vi "check config on connection.vi"() -> (3 "config data out":T18={"Message"={"Parameters"={"FPGA Ref"=refnum, "configID"=0, "activeChannels"=[]}, "Variables"={"RT Status"={"Comms loop"=FALSE, "scheduler loop"=FALSE, "data process loop"=FALSE, "FIFO loop"=FALSE, "Command Stream"=FALSE, "Error Stream"=FALSE, "FPGA FIFO"=FALSE, "Data Stream"=FALSE}, "watchdog"=timestamp(0 s since 1904-01-01), "limitsEnabled"=FALSE, "Interlocks"={"gearboxOil"=FALSE, "bearingOil"=FALSE, "gearboxAir"=FALSE}}}, "FIFO"={"Params"={"FPGA ref"=refnum, "Total Channels"=0}, "Variables"={"FIFO wait counter"=0, "FIFO read trigger"=0}}, "Comms data"={"Parameters"={"error writer name"="", "command reader name"="", "error buffer size"=0, "command buffer size"=0, "scanivalveIP"="", "scanivalvePeriod"=0}, "Variables"={"listen schedule"=0, "incident buffer"=[], "command stream"="", "error stream"="", "waiting for command stream connect"=FALSE, "waiting for error stream connect"=FALSE, "scanivalve connection"=refnum, "scanivalveScheduleID"=0, "activeScanivalvePorts"=[], "channelCount"=0}, "scanivalveConfig"={"listS"={"period"=0, "ADtrig"=FALSE, "ScanTrig"=FALSE, "page"=0, "qpkts"=0}, "listC"={"ZC"=FALSE, "unitScan"="", "CvtUnit"=0.0, "bin"=FALSE, "EU"=FALSE}, "listSG"={"Avg1"=0, "FPS1"=0, "SGEnable1"=FALSE}, "activeChannels"={"Chan1"={"101"=FALSE, "102"=FALSE, "103"=FALSE, "104"=FALSE, "109"=FALSE, "110"=FALSE, "111"=FALSE, "112"=FALSE, "201"=FALSE, "202"=FALSE, "203"=FALSE, "204"=FALSE, "209"=FALSE, "210"=FALSE, "211"=FALSE, "212"=FALSE, "301"=FALSE, "302"=FALSE, "303"=FALSE, "304"=FALSE, "309"=FALSE, "310"=FALSE, "311"=FALSE, "312"=FALSE, "401"=FALSE, "402"=FALSE, "403"=FALSE, "404"=FALSE, "409"=FALSE, "410"=FALSE, "411"=FALSE, "412"=FALSE}}}}, "Data processor"={"Parameters"={"FPGA Ref"=refnum, "data stream"={"data writer name"="error writer", "NS write buffer size"=16, "NS Buffer length"=0}, "FIFO Depth"=0, "Channel controls"={"FIFO channel count"=0, "active indices"=[], "active channels"=0, "channelScaling"=[], "scanivalveCount"=0, "channels"=[]}, "safetyChannels"={"oilP"=0, "airP"=0, "water"=0, "channelLimits"=[]}, "speedChannel"=0, "maxSpeedLimit"=0.0, "Torque"={"fixedOffset"=0.0, "filter"=FALSE, "fallingEdge"=FALSE, "swapEncoders"=FALSE}}, "Variables"={"Intermediary buffer"=[], "buffer position"=0, "write loop counter"=0, "NS write trigger"=0, "NS Connection status"=FALSE, "waiting for NS"=FALSE, "labAmbient"={"pressure"=0.0, "temperature"=0.0}, "scanivalvePorts"=[], "scanivalvePressures"=[], "data stream"="", "activeChannelLimitIndex"=[], "runningSpeedLimit"=0.0, "speedChannelIndex"=0, "Interlocks"={"gearboxOil"=FALSE, "bearingOil"=FALSE, "gearboxAir"=FALSE}, "interlockChannels"={"gearboxOil"=0, "bearingOil"=0, "air"=0}, "limitStates"=[]}}})   [LabVIEW 2018]
uses:
  Type Defs/Message loop data.ctl
  Type Defs/FPGA reference.ctl
  Type Defs/RT Status.ctl
  Type Defs/Analogue loop data.ctl
  Communications loop/comms data.ctl
  Type Defs/generic incident.ctl
  ICL-LabVIEW_General/Scanivalve API project/full interface/polymorphic/scanivalveConfig.ctl
  ICL-LabVIEW_General/Scanivalve API project/full interface/listS.ctl
  ICL-LabVIEW_General/Scanivalve API project/full interface/listC.ctl
  ICL-LabVIEW_General/Scanivalve API project/full interface/listSG.ctl
  ICL-LabVIEW_General/Scanivalve API project/full interface/chan1.ctl
  Type Defs/Data processing loop data.ctl
  PC/type defs/channelControl.ctl
  Type Defs/channelScalingTypes.ctl
  Type Defs/scalingMethods.ctl
  ICL-LabVIEW_General/data channels/parent class/Data Channel.lvclass
  PC/type defs/channelLimitControl.ctl
  PC/type defs/limitActions.ctl
  Type Defs/channelConfigFilePath.ctl
  Type Defs/configFilePath.ctl
  <resource>/objmgr/ni.dex.rc
  ICL-LabVIEW_General/Scanivalve API project/Scanivalve API.lvlib
types:
  T1 = typedef "Message loop data.ctl" = cluster{"Parameters":cluster{"FPGA Ref":T2, "configID":u32, "activeChannels":cluster{"index":u16, "name":string}[]}, "Variables":cluster{"RT Status":T3, "watchdog":timestamp, "limitsEnabled":bool, "Interlocks":cluster{"gearboxOil":bool, "bearingOil":bool, "gearboxAir":bool}}}
  T2 = typedef "FPGA reference.ctl" = refnum<k20>
  T3 = typedef "RT Status.ctl" = cluster{"Comms loop":bool, "scheduler loop":bool, "data process loop":bool, "FIFO loop":bool, "Command Stream":bool, "Error Stream":bool, "FPGA FIFO":bool, "Data Stream":bool}
  T4 = typedef "Analogue loop data.ctl" = cluster{"Params":cluster{"FPGA ref":T2, "Total Channels":u32}, "Variables":cluster{"FIFO wait counter":u16, "FIFO read trigger":u32}}
  T5 = typedef "comms data.ctl" = cluster{"Parameters":cluster{"error writer name":string, "command reader name":string, "error buffer size":i32, "command buffer size":i32, "scanivalveIP":string, "scanivalvePeriod":u16}, "Variables":cluster{"listen schedule":u32, "incident buffer":T6[], "command stream":refnum<k21>, "error stream":refnum<k21>, "waiting for command stream connect":bool, "waiting for error stream connect":bool, "scanivalve connection":refnum<k5>, "scanivalveScheduleID":u32, "activeScanivalvePorts":i32[], "channelCount":i16}, "scanivalveConfig":T7}
  T6 = typedef "generic incident.ctl" = cluster{"timestamp":timestamp, "type":string, "Variant":variant}
  T7 = typedef "Scanivalve API.lvlib/scanivalveConfig.ctl" = cluster{"listS":T8, "listC":T9, "listSG":T10, "activeChannels":T11}
  T8 = typedef "Scanivalve API.lvlib/listS.ctl" = cluster{"period":u16, "ADtrig":bool, "ScanTrig":bool, "page":u16, "qpkts":u16}
  T9 = typedef "Scanivalve API.lvlib/listC.ctl" = cluster{"ZC":bool, "unitScan":string, "CvtUnit":dbl, "bin":bool, "EU":bool}
  T10 = typedef "Scanivalve API.lvlib/listSG.ctl" = cluster{"Avg1":u16, "FPS1":u16, "SGEnable1":bool}
  T11 = typedef "Scanivalve API.lvlib/chan1.ctl" = cluster{"Chan1":cluster{"101":bool, "102":bool, "103":bool, "104":bool, "109":bool, "110":bool, "111":bool, "112":bool, "201":bool, "202":bool, "203":bool, "204":bool, "209":bool, "210":bool, "211":bool, "212":bool, "301":bool, "302":bool, "303":bool, "304":bool, "309":bool, "310":bool, "311":bool, "312":bool, "401":bool, "402":bool, "403":bool, "404":bool, "409":bool, "410":bool, "411":bool, "412":bool}}
  T12 = typedef "Data processing loop data.ctl" = cluster{"Parameters":cluster{"FPGA Ref":T2, "data stream":cluster{"data writer name":string, "NS write buffer size":i32, "NS Buffer length":u32}, "FIFO Depth":u32, "Channel controls":cluster{"FIFO channel count":i32, "active indices":i16[], "active channels":i32, "channelScaling":T13[], "scanivalveCount":i32, "channels":refnum<class "Data Channel.lvclass">[]}, "safetyChannels":cluster{"oilP":u16, "airP":u16, "water":u16, "channelLimits":T16[]}, "speedChannel":i32, "maxSpeedLimit":dbl, "Torque":cluster{"fixedOffset":dbl, "filter":bool, "fallingEdge":bool, "swapEncoders":bool}}, "Variables":cluster{"Intermediary buffer":dbl[][], "buffer position":u32, "write loop counter":u16, "NS write trigger":u32, "NS Connection status":bool, "waiting for NS":bool, "labAmbient":cluster{"pressure":dbl, "temperature":dbl}, "scanivalvePorts":u16[], "scanivalvePressures":dbl[], "data stream":refnum<k21>, "activeChannelLimitIndex":u16[], "runningSpeedLimit":dbl, "speedChannelIndex":i32, "Interlocks":cluster{"gearboxOil":bool, "bearingOil":bool, "gearboxAir":bool}, "interlockChannels":cluster{"gearboxOil":i32, "bearingOil":i32, "air":i32}, "limitStates":cluster{"warn":bool, "alarm":bool}[]}}
  T13 = typedef "channelControl.ctl" = cluster{"index":u16, "active":bool, "channelType":T14, "module":u16, "terminal":u16, "channelName":string, "scalingMethod":T15, "scalingParameters":dbl[], "scaledUnits":string, "tempOffset":dbl}
  T14 = typedef "channelScalingTypes.ctl" = enum16{"calculation", "measurement", "scanivalve", "output", "digital"}
  T15 = typedef "scalingMethods.ctl" = enum16{"none", "linear", "thermocouple", "polynomial", "encoder", "RTD"}
  T16 = typedef "channelLimitControl.ctl" = cluster{"channelID":u16, "Enabled":bool, "warnValue":dbl, "limitValue":dbl, "Invert":bool, "limitAction":T17}
  T17 = typedef "limitActions.ctl" = enum16{"stop", "shutdown", "ignore"}
  T18 = cluster{"Message":T1, "FIFO":T4, "Comms data":T5, "Data processor":T12}
  T19 = typedef "configFilePath.ctl" = path
  T20 = typedef "channelConfigFilePath.ctl" = path
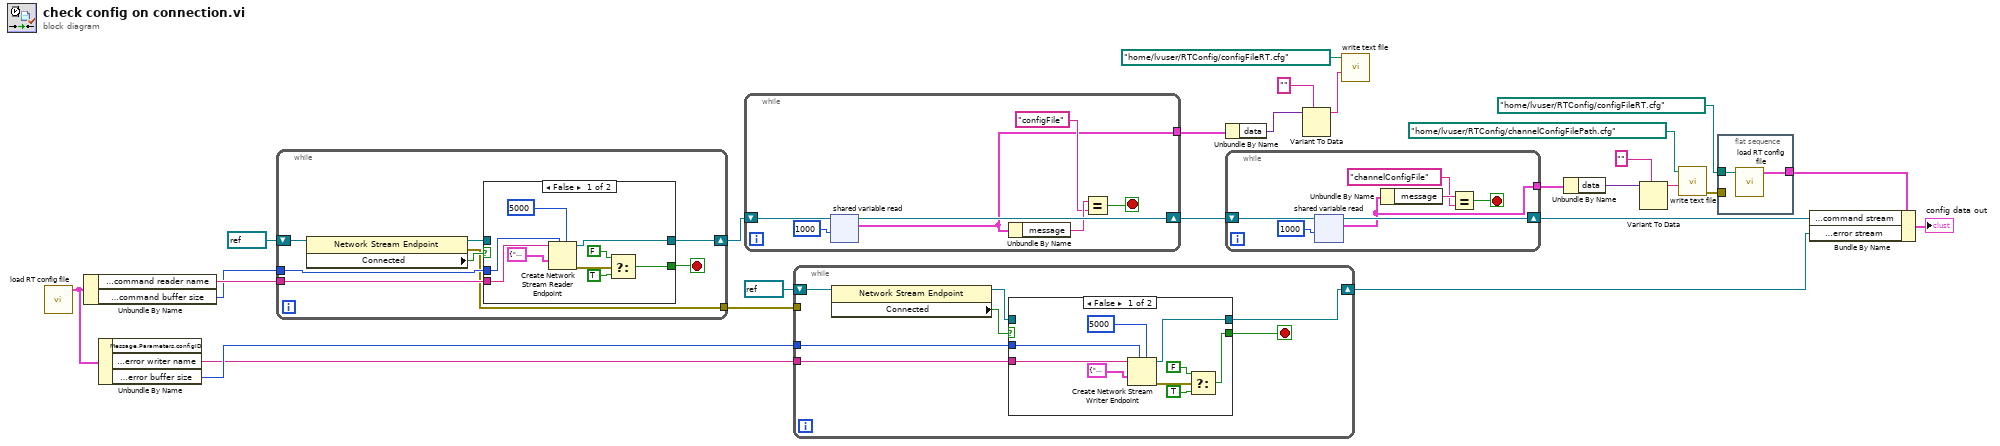
[diagram p0: block diagram]
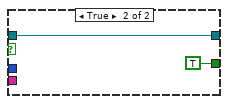
[diagram p3: hidden frame]
diagram:
  n1 = call "load RT config file.vi"() -> ("config data out"=w15:T18)  [unwired: 8 in, 3 out]
  n2 = Unbundle By Name(w15) -> ("Comms data.Parameters.command reader name"=w25:string, "Comms data.Parameters.command buffer size"=w24:i32)
  n3 = Unbundle By Name(w15) -> ("Comms data.Parameters.error writer name"=w20:string, "Comms data.Parameters.error buffer size"=w21:i32)  [unwired: 1 out]
  n4 = while {
    shift-right: [w31] -> w19
    shift-left: refnum<k21> refnum ("Variables.command stream") -> [w34]
    tunnel: w25 -> [w29]
    tunnel: w24 -> [w30]
    tunnel: [w27] -> w23
    stop <- w28 stop-if-true
    n5 = property class="Network Stream Endpoint"(reference=w34) -> (reference out=w32:refnum<k21>, error out=w27:errorcluster, "Connected"=w33:bool)  [unwired: 1 in]
    n6 = case shown="False" w33 {
      tunnel: w32 -> [_ w45]
      tunnel: [w39 w45] -> w31
      tunnel: w30 -> [w42 _]
      tunnel: w29 -> [w40 _]
      tunnel: [w36 TRUE] -> w28
      frame False {
        n7 = Create Network Stream Reader Endpoint(5:5000 ("timeout in ms (-1)"), 7:w42, 9:cluster{"message":string, "data":variant} {"message"="", "data"=variant}, 11:w40) -> (0:w38:errorcluster, 3:w39:refnum<k21>)  [unwired: 3 in]
        n8 = Select(t=FALSE, s=w38, f=TRUE) -> (s? t:f=w36:bool)
      }
      frame True {
      }
    }
  }
  n9 = while {
    shift-right: [w50] -> w16
    shift-left: w19 -> [w52]
    tunnel: [w46] -> w18
    stop <- w47 stop-if-true
    n10 = shared-variable-read(w52, 1000 ("timeout ms (-1)")) -> (w50:refnum<k21>, w46:cluster{"message":string, "data":variant})  [unwired: 1 in, 2 out]
    n11 = Unbundle By Name(w46) -> ("message"=w49:string)
    n12 = Equal?(x=w49, y="configFile") -> (x = y?=w47:bool)
  }
  n13 = while {
    tunnel: w23 -> [_]
    shift-right: [w55] -> w17
    shift-left: refnum<k21> refnum ("writer endpoint") -> [w59]
    tunnel: w21 -> [w57]
    tunnel: w20 -> [w56]
    stop <- w54 stop-if-true
    n14 = property class="Network Stream Endpoint"(reference=w59) -> (reference out=w53:refnum<k21>, "Connected"=w58:bool)  [unwired: 1 in, 1 out]
    n15 = case shown="False" w58 {
      selector: w58 -> [_ w70]
      tunnel: w57 -> [w66 _]
      tunnel: w56 -> [w65 _]
      tunnel: [w64 w69] -> w55
      tunnel: [w60 w70] -> w54
      tunnel: w53 -> [_ w69]
      frame False {
        n16 = Create Network Stream Writer Endpoint(5:5000 ("timeout in ms (-1)"), 7:w66, 9:cluster{"message":string, "data":variant} {"message"="", "data"=variant}, 11:w65) -> (0:w62:errorcluster, 3:w64:refnum<k21>)  [unwired: 3 in]
        n17 = Select(t=FALSE, s=w62, f=TRUE) -> (s? t:f=w60:bool)
      }
      frame True {
      }
    }
  }
  n18 = Unbundle By Name(w18) -> ("data"=w13:variant)
  n19 = while {
    shift-right: [w75] -> w8
    shift-left: w16 -> [w77]
    tunnel: [w71] -> w9
    stop <- w72 stop-if-true
    n20 = shared-variable-read(w77, 1000 ("timeout ms (-1)")) -> (w75:refnum<k21>, w71:cluster{"message":string, "data":variant})  [unwired: 1 in, 2 out]
    n21 = Unbundle By Name(w71) -> ("message"=w74:string)
    n22 = Equal?(x=w74, y="channelConfigFile") -> (x = y?=w72:bool)
  }
  n23 = Variant To Data(type="", Variant=w13) -> (data=w10:string)  [unwired: 1 in, 1 out]
  n24 = call "write text file.vi"("file contents"=w10, "file path"=T19 path "/home/lvuser/RTConfig/configFileRT.cfg" ("file path (use dialog)")) -> ()  [unwired: 9 in, 1 out]
  n25 = Unbundle By Name(w9) -> ("data"=w4:variant)
  n26 = Variant To Data(type="", Variant=w4) -> (data=w6:string)  [unwired: 1 in, 1 out]
  n27 = call "write text file.vi"("file contents"=w6, "file path"=T20 path "/home/lvuser/RTConfig/channelConfigFilePath.cfg" ("channelConfigFilePath")) -> ("error out"=w2:errorcluster)  [unwired: 9 in]
  n28 = flat-sequence {
    tunnel: [w79] -> w7
    tunnel: w2 -> [_]
    tunnel: T19 path "/home/lvuser/RTConfig/configFileRT.cfg" ("file path (use dialog)") -> [w78]
    frame #0 {
      n29 = call "load RT config file.vi"("configuration file path (RT local)"=w78) -> ("config data out"=w79:T18)  [unwired: 7 in, 3 out]
    }
  }
  n30 = Bundle By Name(cluster=w7, "Comms data.Variables.command stream"=w8, "Comms data.Variables.error stream"=w17) -> (→"config data out":T18)
